vi "dashboard.vi"() -> ()   [LabVIEW 2022 SP3]
uses:
  <vilib>/Utility/config.llb/NI_LVConfig.lvlib
panel:
  out "JSON Sent":string
  out "Numeric":i32
  in  "5":bool
  in  "4":bool
  in  "3":bool
  in  "2":bool
  in  "1":bool
  in  "Ignition Safety":bool
  in  "Ignition":bool
  out "WF Chart 1":waveform(dbl)[](graph)
  out "WF Chart 2":waveform(dbl)[](graph)
  out "WF Chart 3":waveform(dbl)[](graph)
  out "WF Chart 4":waveform(dbl)[](graph)
  out "Raw JSON":string
  in  "Port":i32=5005
  in  "Address":string="127.0.0.1"
  out "Current Timestamp":string
  in  "Loop Speed (ms)":i32=10
  out "Command Bytes Written":dbl
  in  "Config File Path":path=path "C:/Users/ajben/OneDrive/Documents/GitHub/labjack/LabVIEW Projects/titan.ini"
  out "String 2":string
  out "Command Sent":string
  out "Console Message":string
  in  "Stop":bool
  # "Switch 1"
  # "Switch 2"
  # "Switch 3"
  # "Switch 4"
  # "Switch 5"
  # "Switch 6"
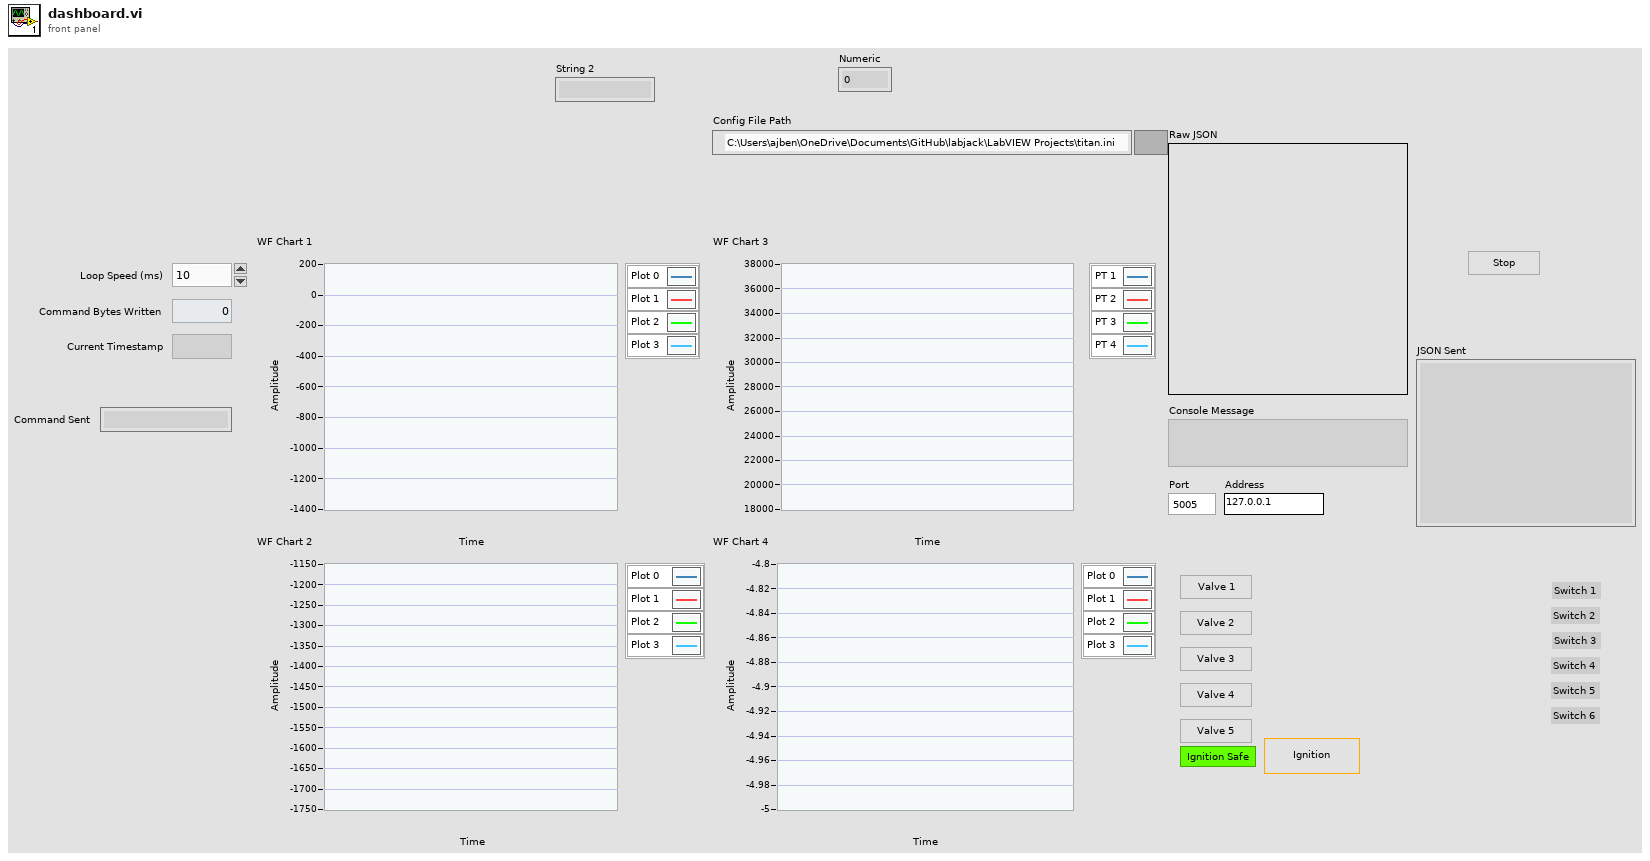
[diagram p1: front panel]
types:
  T1 = cluster{"Chart 1":cluster{"Name":string, "Sensor Names":string[], "Sensors":i32[]}, "Chart 2":cluster{"Name":string, "Sensor Names":string[], "Sensors":i32[]}, "Chart 3":cluster{"Name":string, "Sensor Names":string[], "Sensors":i32[]}, "Chart 4":cluster{"Name":string, "Sensor Names":string[], "Sensors":i32[]}}
  T2 = cluster{"states":i32[], "timestamp":string, "console":string, "sensors":dbl[]}
  T3 = cluster{"command":string, "driver":i32, "value":i32}
  T4 = typedef "eventsource.ctl" = u32
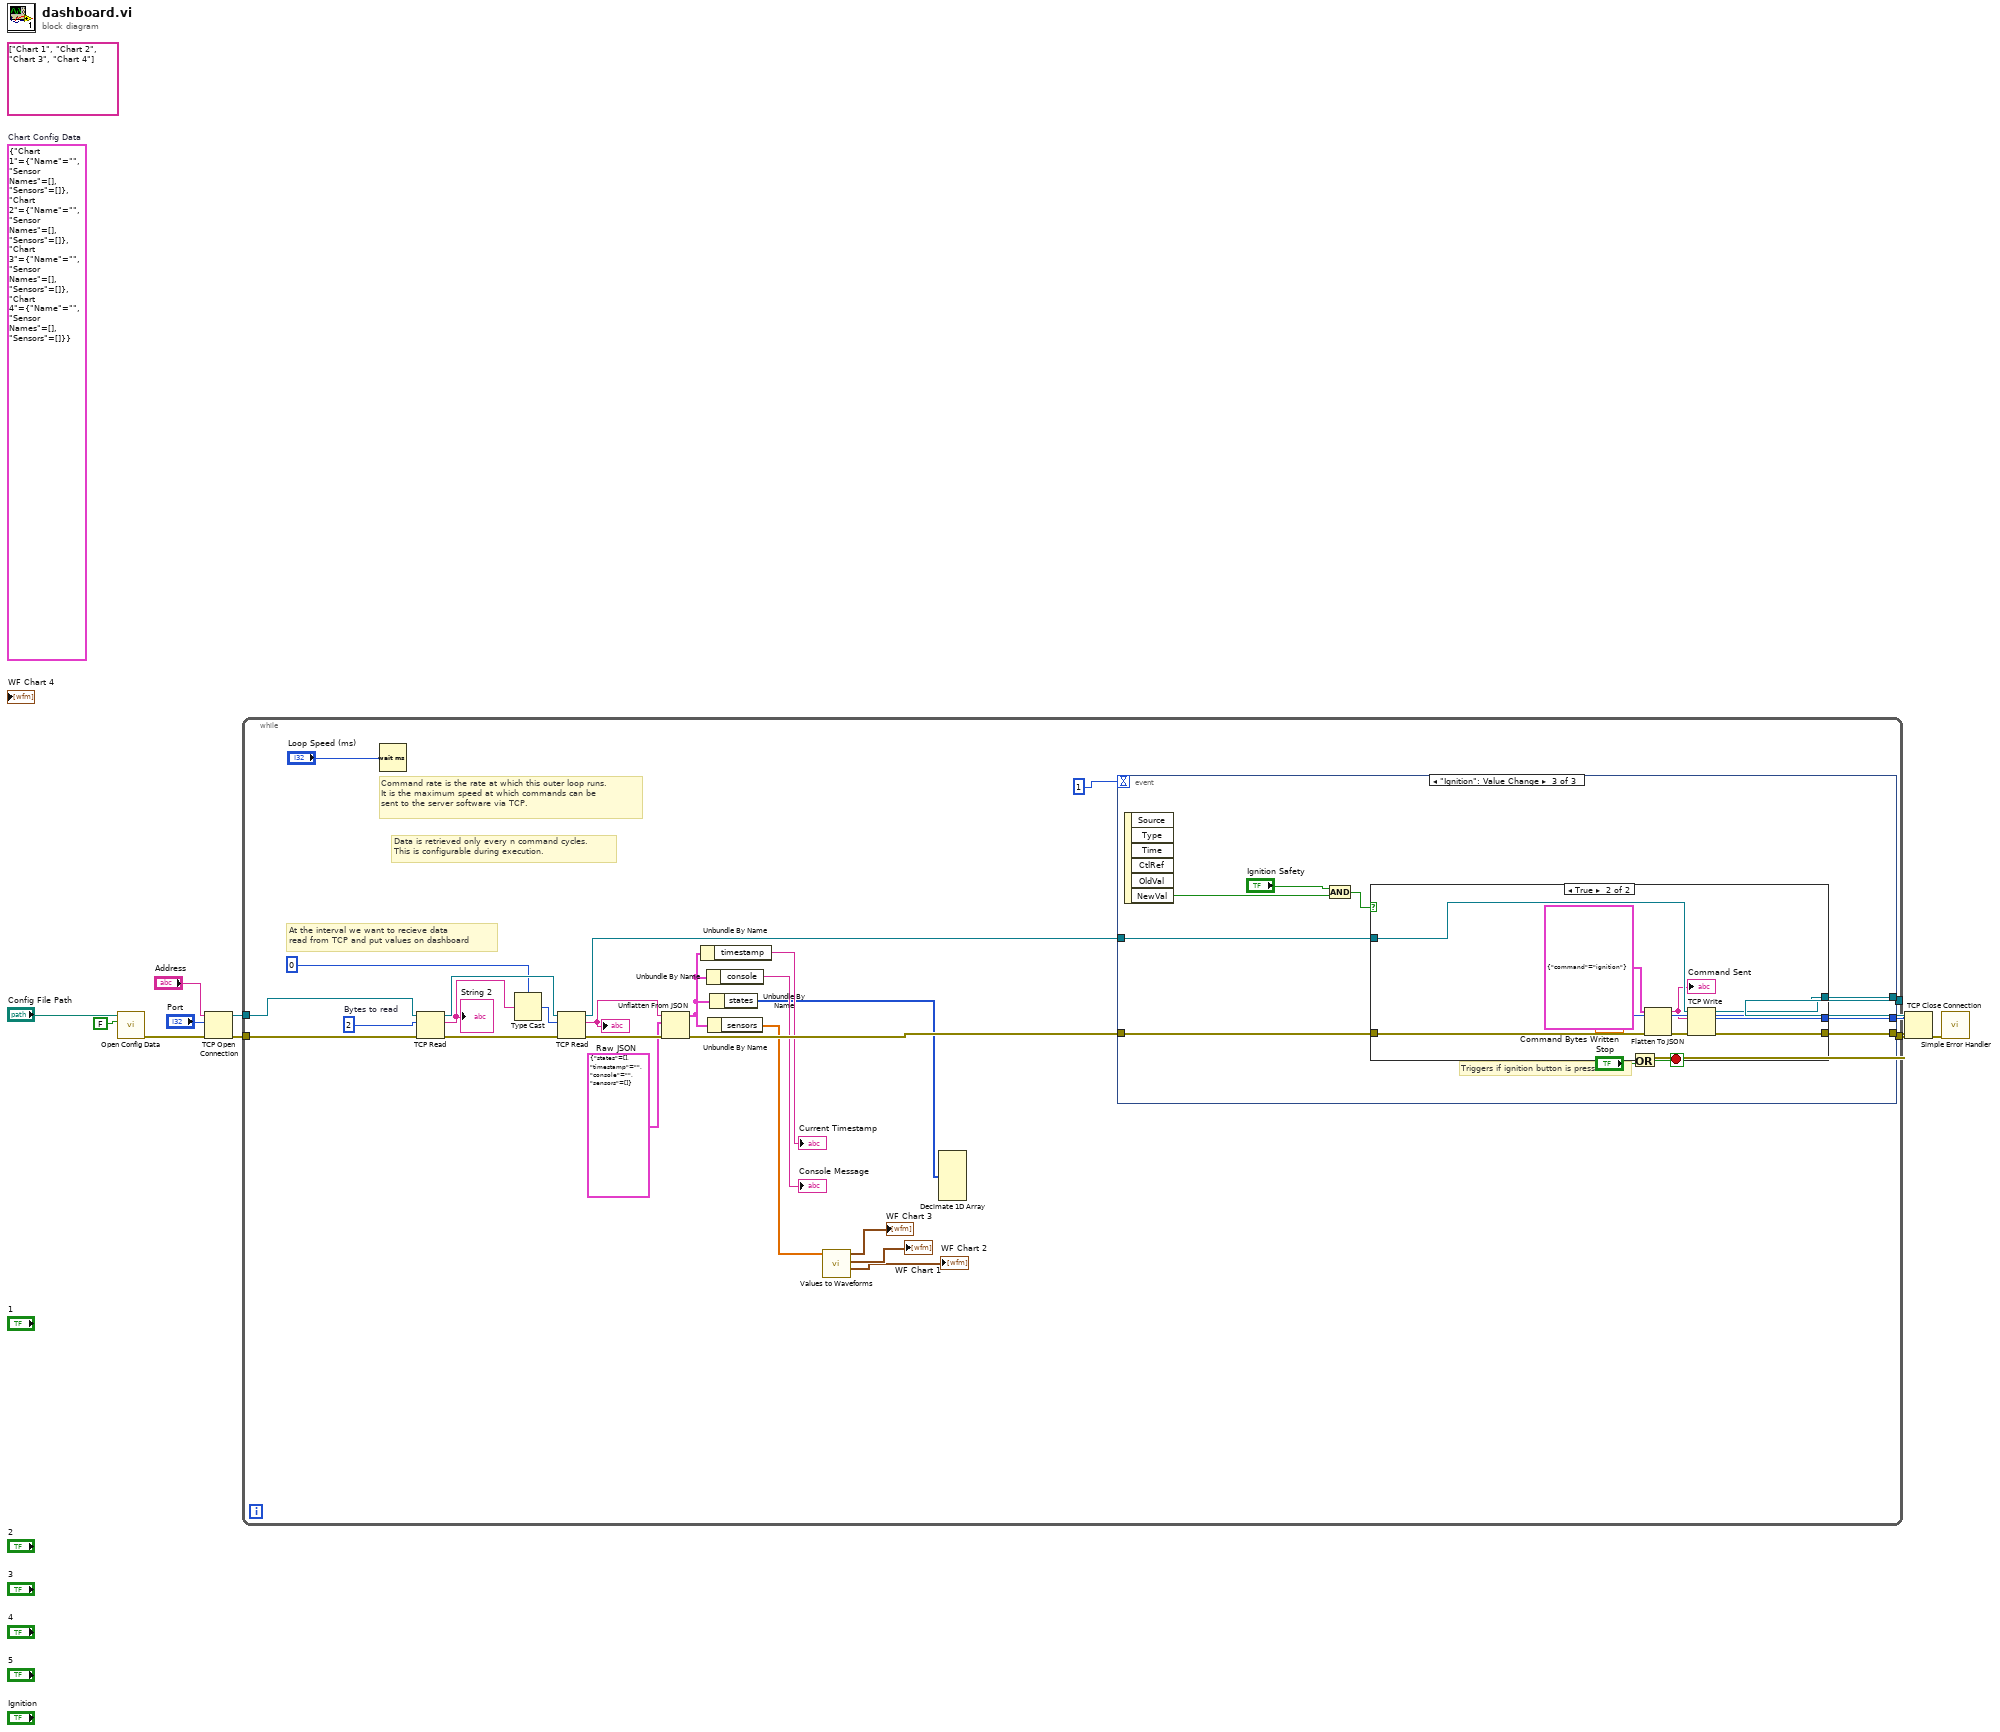
[diagram p0: block diagram]
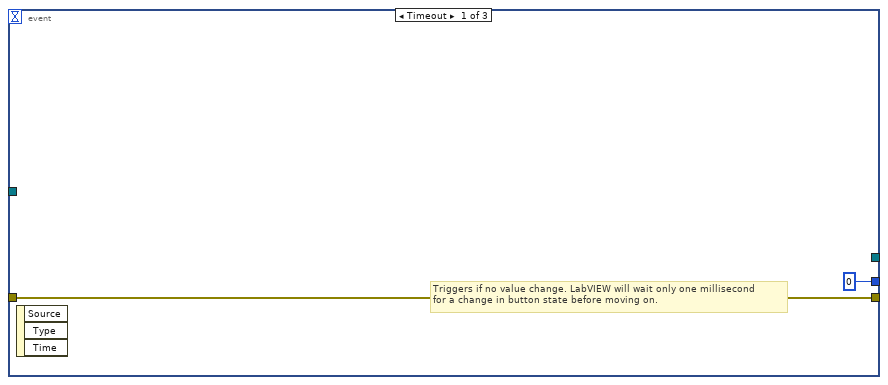
[diagram p2: hidden frame]
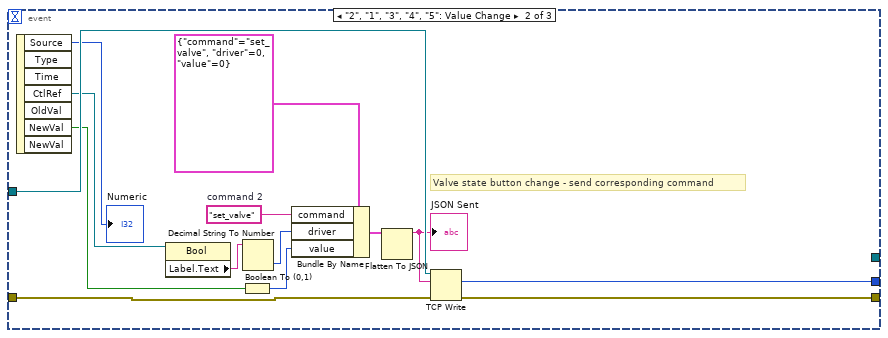
[diagram p3: hidden frame]
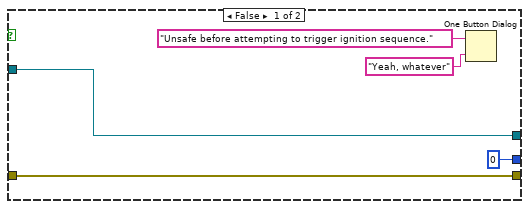
[diagram p4: hidden frame]
diagram:
  (unwired) string[] ["Chart 1", "Chart 2", "Chart 3", "Chart 4"]
  (unwired) T1 {"Chart 1"={"Name"="", "Sensor Names"=[], "Sensors"=[]}, "Chart 2"={"Name"="", "Sensor Names"=[], "Sensors"=[]}, "Chart 3"={"Name"="", "Sensor Names"=[], "Sensors"=[]}, "Chart 4"={"Name"="", "Sensor Names"=[], "Sensors"=[]}}  # Chart Config Data
  n1 = call <vilib>:"Open Config Data.vi"("create file if necessary (T)"=FALSE, "configuration file path"="Config File Path") -> ("error out"=w4:errorcluster)  [unwired: 7 in, 2 out]
  n2 = TCP Open Connection(address="Address", remote port or service name="Port", error in (no error)=w4) -> (connection ID=w9:refnum<k5>, error out=w10:errorcluster)  [unwired: 2 in]
  n3 = while {
    tunnel: w10 -> [w38]
    tunnel: w9 -> [w37]
    tunnel: [w31] -> w3
    tunnel: [w28] -> w1
    stop <- w36 stop-if-true
    w27 = 2  # Bytes to read
    # "At the interval we want to recieve data\nread from TCP and put values on dashboard"
    # "Data is retrieved only every n command cycles.\nThis is configurable during execution."
    # "Command rate is the rate at which this outer loop runs.\nIt is the maximum speed at which commands can be\nsent to the server software via TCP."
    n4 = Wait (ms)(milliseconds to wait="Loop Speed (ms)") -> ()  [unwired: 1 out]
    n5 = TCP Read(connection ID=w37, bytes to read=w27, error in (no error)=w38) -> (connection ID out=w26:refnum<k5>, data out=w12:string, error out=w25:errorcluster)  [unwired: 2 in]
    "String 2" <- w12
    n6 = Type Cast(type=u16 0, x=w12) -> (*(type *) &x=w23:u16)
    n7 = TCP Read(connection ID=w26, bytes to read=w23, error in (no error)=w25) -> (connection ID out=w33:refnum<k5>, data out=w22:string, error out=w21:errorcluster)  [unwired: 2 in]
    "Raw JSON" <- w22
    n8 = Unflatten From JSON(JSON string=w22, type and defaults=T2 {"states"=[], "timestamp"="", "console"="", "sensors"=[]}, error in (no error)=w21) -> (value=w18:T2, error out=w32:errorcluster)  [unwired: 4 in]
    n9 = Unbundle By Name(w18) -> ("timestamp"=→"Current Timestamp":string)
    n10 = Unbundle By Name(w18) -> ("console"=→"Console Message":string)
    n11 = Unbundle By Name(w18) -> ("sensors"=w16:dbl[])
    n12 = Unbundle By Name(w18) -> ("states"=w11:i32[])
    n13 = call "Values to Waveforms.vi"("sensorValues"=w16) -> ("Pressure Transducers"=→"WF Chart 2":waveform(dbl)[], "Temperature"=→"WF Chart 1":waveform(dbl)[], "Load Cells"=→"WF Chart 3":waveform(dbl)[])  [unwired: 8 in]
    n14 = Decimate 1D Array(w11) -> ()  [unwired: 7 out]
    n15 = event shown="[2] \"Ignition\": Value Change" {
      selector: _ -> [_ _ _]
      dyn-events: _ -> [_ _ _]
      timeout: 1 -> [_ _ _]
      tunnel: w33 -> [_ w52 w59]
      tunnel: [w40 w54 w61] -> w31
      tunnel: w32 -> [w40 w53 w62]
      tunnel: [0 w46 w60] -> w29
      tunnel: [_ _ w55] -> w28
      event Timeout {
        # "Triggers if no value change. LabVIEW will wait only one millisecond\nfor a change in button state before moving on."
        n16 = event-data() -> ()  [unwired: 1 in, 3 out]
      }
      event "2", "1", "3", "4", "5": Value Change {
        w47 = "set_valve"  # command 2
        # "Valve state button change - send corresponding command"
        n17 = event-data() -> ("Source"=→"Numeric":T4, "CtlRef"=w44:refnum<vi>, "NewVal"=w51:bool)  [unwired: 1 in, 4 out]
        n18 = property class="Bool"(reference=w44) -> ("Label.Text"=w42:string)  [unwired: 1 in, 2 out]
        n19 = Boolean To (0,1)(Boolean=w51) -> (0, 1=w49:i16)
        n20 = Decimal String To Number(string=w42) -> (number=w41:i32)  [unwired: 2 in, 1 out]
        n21 = Bundle By Name(cluster=T3 {"command"="set_valve", "driver"=0, "value"=0}, "command"=w47, "driver"=w41, "value"=w49) -> (w48:T3)
        n22 = Flatten To JSON(anything=w48) -> (JSON string=w43:string)  [unwired: 2 in, 1 out]
        "JSON Sent" <- w43
        n23 = TCP Write(connection ID=w52, data in=w43, error in (no error)=w53) -> (bytes written=w46:i32, error out=w54:errorcluster)  [unwired: 1 in, 1 out]
      }
      event "Ignition": Value Change {
        # "Triggers if ignition button is pressed"
        n24 = event-data() -> ("NewVal"=w56:bool)  [unwired: 1 in, 5 out]
        n25 = And(x="Ignition Safety", y=w56) -> (x .and. y?=w58:bool)
        n26 = case shown="True" w58 {
          tunnel: w62 -> [w67 w74]
          tunnel: [w67 w72] -> w61
          tunnel: [0 w71] -> w60
          tunnel: w59 -> [w63 w70]
          tunnel: [w63 w68] -> w55
          frame False {
            n27 = One Button Dialog(message="Unsafe before attempting to trigger ignition sequence.", button name ("OK")="Yeah, whatever") -> ()  [unwired: 1 out]
          }
          frame True {
            n28 = Flatten To JSON(anything=cluster{"command":string} {"command"="ignition"}, error in (no error)=w74) -> (JSON string=w69:string, 11:w73:errorcluster)  [unwired: 1 in]
            "Command Sent" <- w69
            n29 = TCP Write(connection ID=w70, data in=w69, error in (no error)=w73) -> (connection ID out=w68:refnum<k5>, bytes written=w71:i32, error out=w72:errorcluster)  [unwired: 1 in]
          }
        }
      }
    }
    "Command Bytes Written" <- w29
    n30 = Or(x=w31, y="Stop") -> (x .or. y?=w36:bool)
  }
  n31 = TCP Close Connection(connection ID=w1, error in (no error)=w3) -> (error out=w2:errorcluster)  [unwired: 1 in, 1 out]
  n32 = call <vilib>:"Simple Error Handler.vi"("error in (no error)"=w2) -> ()  [unwired: 4 in, 5 out]
